vi "WriteSLMPAttern.vi"(8 "Holo Array":T1[](array[typedef]) {"Modes"."Amplititute" step=0.05}, 11 "General settings":T2) -> (3 "Display Array":u8[][](array[numeric]))   [LabVIEW 2014]
uses:
  Controls/SLM General Settings.ctl
  Controls/Holo Controls.ctl
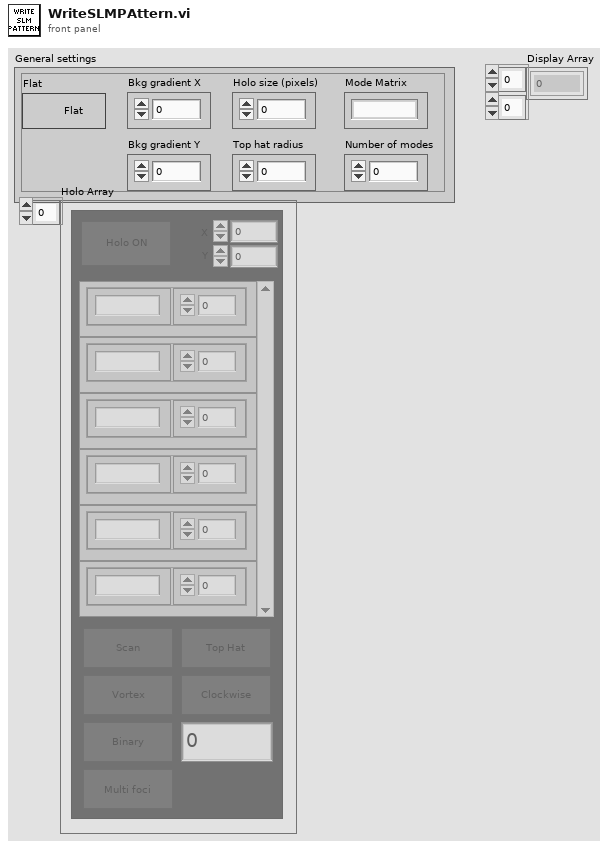
[diagram p1: front panel]
types:
  T1 = typedef "Holo Controls.ctl" = cluster{"Top Hat":bool, "Modes":cluster{"Mode ID":string, "Amplititute":dbl}[], "Vortex":bool, "Clockwise":bool, "X":dbl, "Y":dbl, "Holo ON":bool, "Scan":bool, "Binary":bool, "Binary Angle":dbl, "Multi foci":bool}
  T2 = typedef "SLM General Settings.ctl" = cluster{"Holo size (pixels)":i32, "Top hat radius":dbl, "Number of modes":i32, "Bkg gradient X":dbl, "Bkg gradient Y":dbl, "Flat":bool, "Mode Matrix":u16}
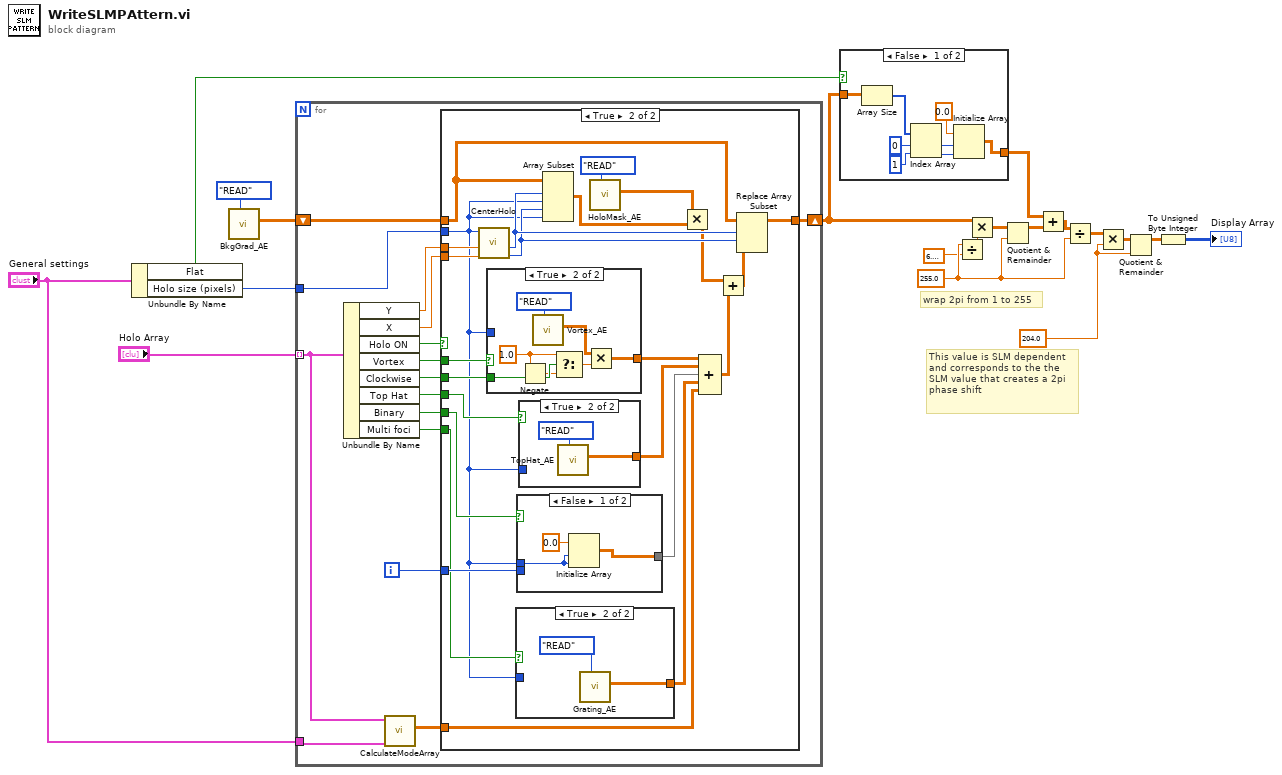
[diagram p0: block diagram]
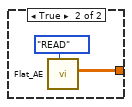
[diagram p2: hidden frame]
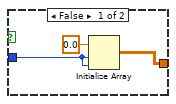
[diagram p4: hidden frame]
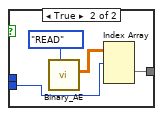
[diagram p5: hidden frame]
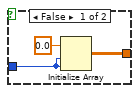
[diagram p6: hidden frame]
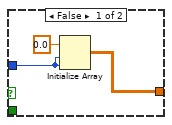
[diagram p7: hidden frame]
diagram:
  w19 = 204.0 ("Wrap Value")
  w13 = 255.0 ("y")
  # "This value is SLM dependent and corresponds to the the SLM value that creates a 2pi phase shift"
  # "wrap 2pi from 1 to 255"
  n1 = Unbundle By Name("General settings") -> ("Flat"=w9:bool, "Holo size (pixels)"=w1:i32)
  n2 = call "BkgGrad_AE.vi"("Action"=enum16{"READ", "WRITE"}."READ") -> ("BkgGrad Out"=w5:dbl[][])  [unwired: 10 in]
  n3 = for {
    tunnel: "Holo Array" -> [w24] mode=indexing
    tunnel: w1 -> [w30]
    shift-right: [w26] -> w2
    shift-left: w5 -> [w27]
    tunnel: "General settings" -> [w23]
    i -> [w21]
    n4 = Unbundle By Name(w24) -> ("Y"=w29:dbl, "X"=w28:dbl, "Holo ON"=w31:bool, "Vortex"=w34:bool, "Clockwise"=w33:bool, "Top Hat"=w32:bool, "Binary"=w22:bool, "Multi foci"=w20:bool)
    n5 = call "CalculateModeArray.vi"("General settings"=w23, "Holo Control"=w24) -> ("ModeArray"=w25:dbl[][])  [unwired: 9 in]
    n6 = case shown="True" w31 {
      tunnel: w34 -> [_ w55]
      tunnel: w33 -> [_ w59]
      tunnel: w27 -> [w35 w51]
      tunnel: w32 -> [_ w54]
      tunnel: w30 -> [_ w36]
      tunnel: w29 -> [_ w58]
      tunnel: w28 -> [_ w57]
      tunnel: [w35 w52] -> w26
      tunnel: w25 -> [_ w39]
      tunnel: w22 -> [_ w42]
      tunnel: w21 -> [_ w40]
      tunnel: w20 -> [_ w38]
      frame False {
      }
      frame True {
        n7 = call "CenterHolo.vi"("X"=w57, "Y"=w58, "Holo Size"=w36) -> ("X centered"=w49:i32, "Y centered"=w50:i32)  [unwired: 7 in]
        n8 = case shown="True" w55 {
          tunnel: w59 -> [_ w86]
          tunnel: [w78 w80] -> w48
          tunnel: w36 -> [w77 _]
          frame False {
            n9 = Initialize Array(0.0 ("element"), w77, w77) -> (w78:dbl[][])
          }
          frame True {
            w85 = 1.0 ("t")
            n10 = Negate(x=w85) -> (-x=w84:dbl)
            n11 = call "Vortex_AE.vi"("Action"=enum16{"READ", "WRITE"}."READ") -> ("Vortex Out"=w82:dbl[][])  [unwired: 10 in]
            n12 = Select(t=w85, s=w86, f=w84) -> (s? t:f=w81:dbl)
            n13 = Multiply(x=w82, y=w81) -> (x*y=w80:dbl[][])
          }
        }
        n14 = case shown="True" w38 {
          tunnel: [w61 w63] -> w37
          tunnel: w36 -> [w60 _]
          frame False {
            n15 = Initialize Array(0.0 ("element"), w60, w60) -> (w61:dbl[][])
          }
          frame True {
            n16 = call "Grating_AE.vi"("Action"=enum16{"READ", "WRITE"}."READ") -> ("Grating Out"=w63:dbl[][])  [unwired: 10 in]
          }
        }
        n17 = case shown="False" w42 {
          tunnel: [w66 w69] -> w41
          tunnel: w36 -> [w65 _]
          tunnel: w40 -> [_ w68]
          frame False {
            n18 = Initialize Array(0.0 ("element"), w65, w65) -> (w66:dbl[][])
          }
          frame True {
            n19 = call "Binary_AE.vi"("Action"=enum16{"READ", "WRITE"}."READ") -> ("BINARY Out"=w70:dbl[][][])  [unwired: 10 in]
            n20 = Index Array(array=w70, index (dim 0)=w68) -> (element=w69:dbl[][])  [unwired: 2 in]
          }
        }
        n21 = case shown="True" w54 {
          tunnel: [w73 w75] -> w53
          tunnel: w36 -> [w72 _]
          frame False {
            n22 = Initialize Array(0.0 ("element"), w72, w72) -> (w73:dbl[][])
          }
          frame True {
            n23 = call "TopHat_AE.vi"("Action"=enum16{"READ", "WRITE"}."READ") -> ("TopHat Out"=w75:dbl[][])  [unwired: 10 in]
          }
        }
        n24 = Array Subset(array=w51, index (row)=w50, length (row)=w36, index (col)=w49, length (col)=w36) -> (w43:dbl[][])
        n25 = call "HoloMask_AE.vi"("Action"=enum16{"READ", "WRITE"}."READ") -> ("HoloMask Out"=w44:dbl[][])  [unwired: 10 in]
        n26 = Multiply(x=w44, y=w43) -> (x*y=w47:dbl[][])
        n27 = Compound Arithmetic op=ADD(w48, w53, w41, w37, w39) -> (w45:dbl[][])
        n28 = Add(x=w47, y=w45) -> (x+y=w46:dbl[][])
        n29 = Replace Array Subset(array=w51, new element=w46, index (row)=w50, index (col)=w49) -> (w52:dbl[][])
      }
    }
  }
  n30 = case shown="False" w9 {
    tunnel: [w87 w95] -> w11
    tunnel: w2 -> [w88 _]
    frame False {
      n31 = Array Size(array=w88) -> (size(s)=w90:i32[])
      n32 = Index Array(array=w90, index #1=0 ("index"), index #2=1 ("index")) -> (element #1=w92:i32, element #2=w93:i32)
      n33 = Initialize Array(0.0 ("element"), w92, w93) -> (w87:dbl[][])
    }
    frame True {
      n34 = call "Flat_AE.vi"("Action"=enum16{"READ", "WRITE"}."READ") -> ("Flat Out"=w95:dbl[][])  [unwired: 10 in]
    }
  }
  n35 = Divide(x=w13, y=6.283185307179586) -> (x/y=w7:dbl)
  n36 = Multiply(x=w2, y=w7) -> (x*y=w6:dbl[][])
  n37 = Quotient & Remainder(x=w6, y=w13) -> (x-y*floor(x/y)=w10:dbl[][])  [unwired: 1 out]
  n38 = Add(x=w11, y=w10) -> (x+y=w12:dbl[][])
  n39 = Divide(x=w12, y=w13) -> (x/y=w14:dbl[][])
  n40 = Multiply(x=w14, y=w19) -> (x*y=w15:dbl[][])
  n41 = Quotient & Remainder(x=w15, y=w19) -> (x-y*floor(x/y)=w16:dbl[][])  [unwired: 1 out]
  n42 = To Unsigned Byte Integer(number=w16) -> (unsigned 8bit integer=→"Display Array":u8[][])
